vi "Post Install Action.vi"(10 "Variant":variant) -> (0 "error out":errorcluster)   [LabVIEW 2015]
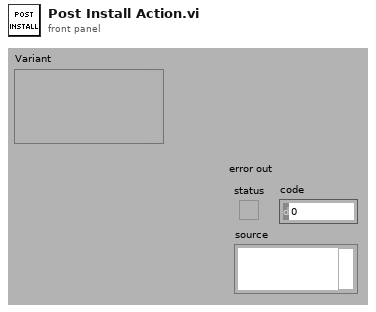
[diagram p1: front panel]
types:
  T1 = typedef "PL_class cache.lvlib/cache definition.ctl" = cluster{"configuration":T2, "class cache data":T3}
  T2 = typedef "PL_class cache.lvlib/cache search configuration.ctl" = cluster{"Search Paths":path[], "Folders to Exclude":string[], "full class list":path[]}
  T3 = typedef "PL_class cache.lvlib/cached class information.ctl" = cluster{"targets":T4[], "engines":T5[], "modules":T5[], "ignored class list":path[]}
  T4 = typedef "PL_class cache.lvlib/target class metadata.ctl" = cluster{"file name":string, "fully qualified name":string, "menu display name":string, "configuration class name":string}
  T5 = typedef "PL_class cache.lvlib/class metadata.ctl" = cluster{"file name":string, "fully qualified name":string, "menu display name":string, "configuration class":string, "category":string, "instances allowed":i32, "supported targets":T6[]}
  T6 = typedef "TBM configuration.lvclass/Target Types.ctl" = enum16{"Windows", "Mac", "Linux", "Linux RT ARM", "VxWorks", "Pharlap", "Other", "Linux RT x64"}
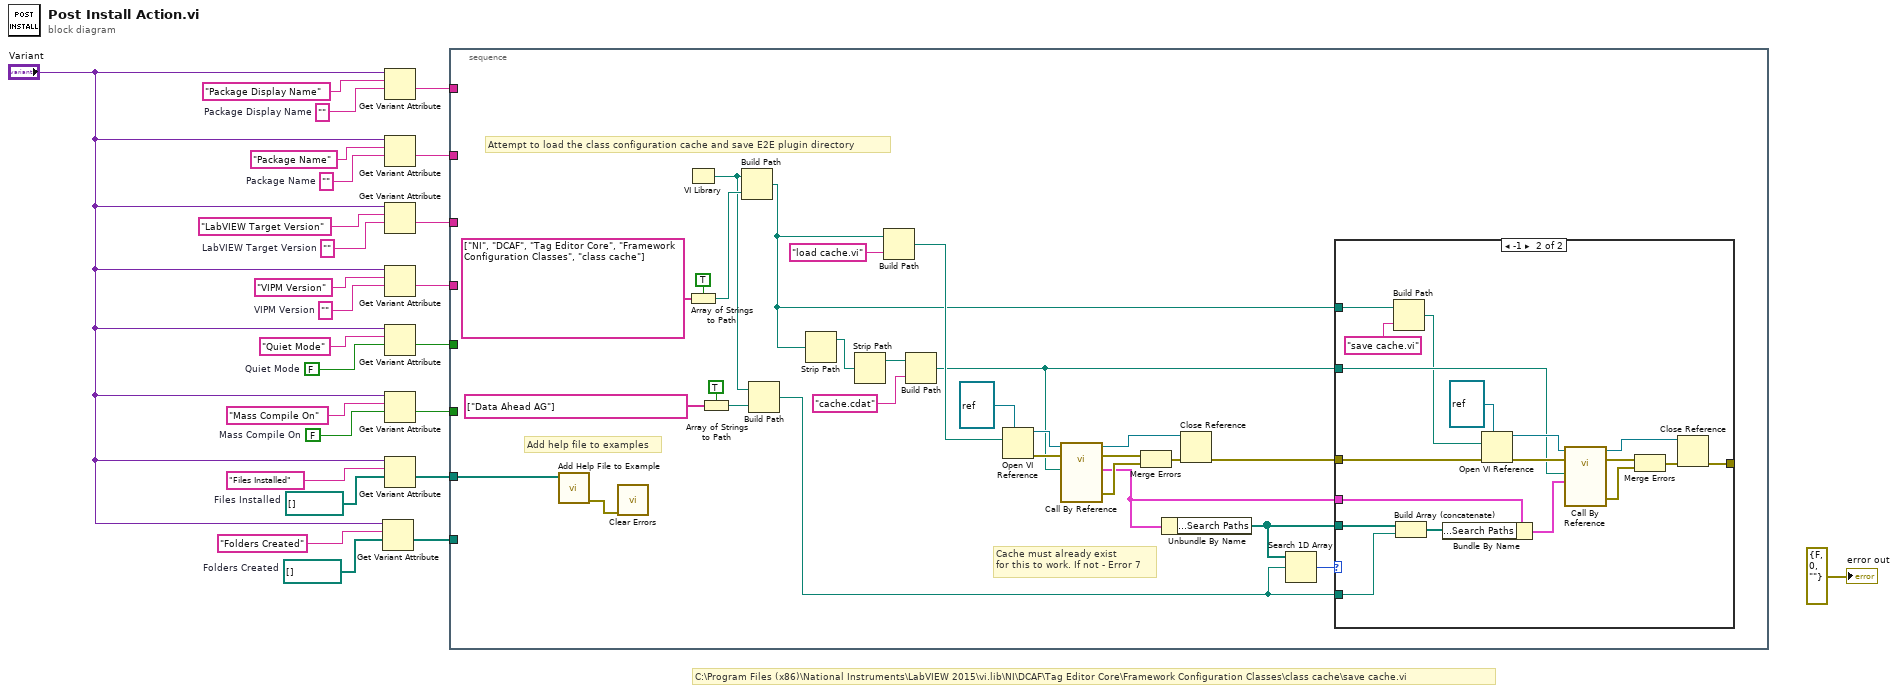
[diagram p0: block diagram]
diagram:
  w1 = path[] []  # Folders Created
  w2 = path[] []  # Files Installed
  w8 = FALSE  # Mass Compile On
  w9 = ""  # Package Display Name
  w16 = FALSE  # Quiet Mode
  w19 = ""  # VIPM Version
  w21 = ""  # LabVIEW Target Version
  w23 = ""  # Package Name
  # "C:\\Program Files (x86)\\National Instruments\\LabVIEW 2015\\vi.lib\\NI\\DCAF\\Tag Editor Core\\Framework Configuration Classes\\class cache\\save cache.vi"
  n1 = Get Variant Attribute(Variant="Variant", name="Folders Created", default value (empty Variant)=w1) -> (value=w6:path[])  [unwired: 1 in, 3 out]
  n2 = Get Variant Attribute(Variant="Variant", name="Package Display Name", default value (empty Variant)=w9) -> (value=w15:string)  [unwired: 1 in, 3 out]
  n3 = Get Variant Attribute(Variant="Variant", name="Package Name", default value (empty Variant)=w23) -> (value=w14:string)  [unwired: 1 in, 3 out]
  n4 = Get Variant Attribute(Variant="Variant", name="LabVIEW Target Version", default value (empty Variant)=w21) -> (value=w13:string)  [unwired: 1 in, 3 out]
  n5 = Get Variant Attribute(Variant="Variant", name="VIPM Version", default value (empty Variant)=w19) -> (value=w12:string)  [unwired: 1 in, 3 out]
  n6 = Get Variant Attribute(Variant="Variant", name="Quiet Mode", default value (empty Variant)=w16) -> (value=w11:bool)  [unwired: 1 in, 3 out]
  n7 = Get Variant Attribute(Variant="Variant", name="Mass Compile On", default value (empty Variant)=w8) -> (value=w10:bool)  [unwired: 1 in, 3 out]
  n8 = Get Variant Attribute(Variant="Variant", name="Files Installed", default value (empty Variant)=w2) -> (value=w5:path[])  [unwired: 1 in, 3 out]
  n9 = stacked-sequence {
    tunnel: w15 -> [_]
    tunnel: w14 -> [_]
    tunnel: w13 -> [_]
    tunnel: w12 -> [_]
    tunnel: w11 -> [_]
    tunnel: w10 -> [_]
    tunnel: w5 -> [w28]
    tunnel: w6 -> [_]
    frame #0 {
      # "Add help file to examples"
      # "Cache must already exist\nfor this to work. If not - Error 7"
      # "Attempt to load the class configuration cache and save E2E plugin directory"
      n10 = call "Add Help File to Example.vi"("Files Installed"=w28) -> ("error out"=w27:errorcluster)  [unwired: 10 in]
      n11 = call <vilib>:"Clear Errors.vi"("error in (no error)"=w27) -> ()  [unwired: 5 in, 2 out]
      n12 = VI Library() -> (path=w29:path)
      n13 = Array of Strings to Path(0:string[] ["NI", "DCAF", "Tag Editor Core", "Framework Configuration Classes", "class cache"], 1:TRUE ("relative")) -> (2:w52:path)
      n14 = Array of Strings to Path(0:string[] ["Data Ahead AG"], 1:TRUE ("relative")) -> (2:w31:path)
      n15 = Build Path(base path=w29, name or relative path=w52) -> (appended path=w34:path)
      n16 = Build Path(base path=w29, name or relative path=w31) -> (appended path=w30:path)
      n17 = Strip Path(path=w34) -> (stripped path=w46:path)  [unwired: 1 out]
      n18 = Strip Path(path=w46) -> (stripped path=w45:path)  [unwired: 1 out]
      n19 = Build Path(base path=w34, name or relative path="load cache.vi") -> (appended path=w49:path)
      n20 = Build Path(base path=w45, name or relative path="cache.cdat") -> (appended path=w35:path)
      n21 = Open VI Reference(type specifier VI Refnum (for type only)=refnum<vi> refnum, vi path=w49) -> (vi reference=w47:refnum<vi>, error out=w48:errorcluster)  [unwired: 4 in]
      n22 = call-by-ref "?"(reference=w47, error in=w48, "cache path"=w35) -> (reference out=w40:refnum<vi>, error out=w43:errorcluster, 0:"error out"=w42:errorcluster, "cache"=w37:T1)  [unwired: 9 in]
      n23 = Merge Errors(w43, w42) -> (w41:errorcluster)
      n24 = Unbundle By Name(w37) -> ("configuration.Search Paths"=w38:path[])
      n25 = Close Reference(reference=w40, error in (no error)=w41) -> (error out=w36:errorcluster)
      n26 = Search 1D Array(1D array=w38, element=w30) -> (index of element=w39:i32)  [unwired: 1 in]
      n27 = case shown="-1" w39 {
        tunnel: w38 -> [_ w73]
        tunnel: w37 -> [_ w71]
        tunnel: w36 -> [w55 w69]
        tunnel: w35 -> [_ w65]
        tunnel: w34 -> [_ w63]
        tunnel: w30 -> [_ w57]
        tunnel: [w55 w56] -> _
        frame Default {
        }
        frame -1 {
          n28 = Build Path(base path=w63, name or relative path="save cache.vi") -> (appended path=w62:path)
          n29 = Build Array (concatenate)(w73, w57) -> (w72:path[])
          n30 = Bundle By Name(cluster=w71, "configuration.Search Paths"=w72) -> (w66:T1)
          n31 = Open VI Reference(type specifier VI Refnum (for type only)=refnum<vi> refnum, vi path=w62, error in (no error)=w69) -> (vi reference=w67:refnum<vi>, error out=w68:errorcluster)  [unwired: 3 in]
          n32 = call-by-ref "?"(reference=w67, error in=w68, "cache"=w66, "path"=w65) -> (reference out=w58:refnum<vi>, error out=w61:errorcluster, 0:"error out"=w60:errorcluster)  [unwired: 9 in]
          n33 = Merge Errors(w61, w60) -> (w59:errorcluster)
          n34 = Close Reference(reference=w58, error in (no error)=w59) -> (error out=w56:errorcluster)
        }
      }
    }
  }
  "error out" <- errorcluster {"status"=FALSE, "code"=0, "source"=""} ("error out")
